vi "CODCr启动 (子VI).vi"(11 "元素":T1(ring)) -> (0 "error out":T2={"status"=FALSE, "代码"=4, "source"=""} caption="错误输出" {"代码" items=["执行成功"=1, "执行失败，但不知道原因"=2, "命令请求条件错误"=3, "通讯超时"=4, "系统繁忙不能执行"=5, "系统故障"=6, "没有数据"=100]})   [LabVIEW 2016]
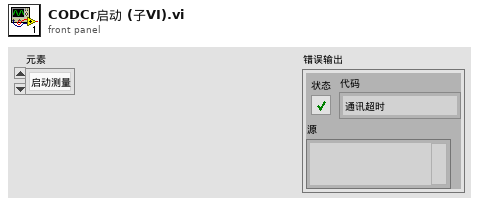
[diagram p1: front panel]
types:
  T1 = enum16{"启动测量", "标样核查", "零点核查", "跨度核查", "空白测试", "平行样测试", "加标回收", "空白校准", "标样校准", "初始化（清洗）", "停止测试", "仪器重启", "校时", "模式设置", "测量间隔设置"}
  T2 = cluster{"status":bool, "代码":u16, "source":string}
  T3 = cluster{"系统时间":timestamp, "工作状态":u16, "测量模式":u16, "告警代码":u16, "故障代码":u16, "日志代码":u16, "软件版本":u16, "F0":sgl, "F1":sgl, "F2":sgl, "F3":sgl, "T":sgl, "H":sgl, "id":u16, "flowid":u16, "量程":u16}
  T4 = cluster{"测量模式":enum16{"水样测量", "标样核查", "零点核查", "跨度核查", "空白测试", "加标回收", "平行样", "校零", "校标"}}
  T5 = enum16{"空闲", "水样测试", "标样核查", "零点核查", "跨度核查", "空白测试", "平行样测试", "加标回收", "空白校准", "标样校准", "初始化（清洗）"}
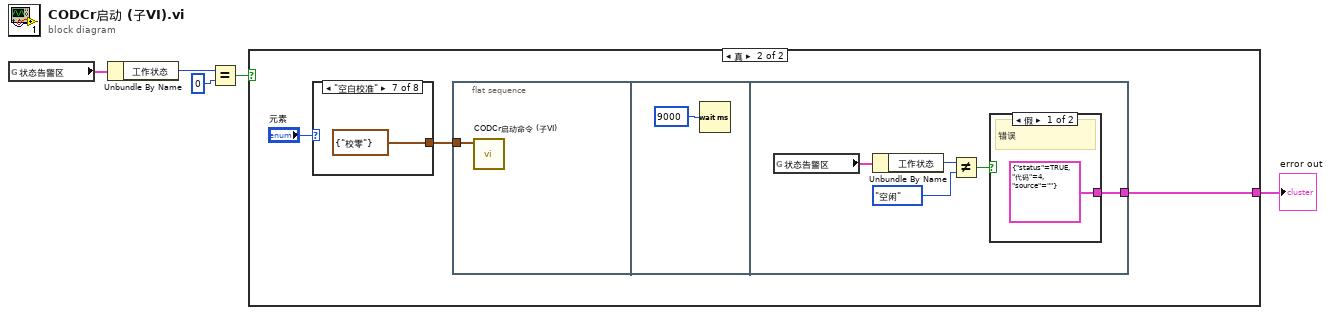
[diagram p0: block diagram]
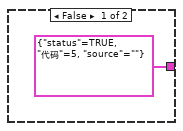
[diagram p2: hidden frame]
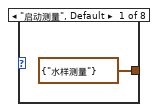
[diagram p3: hidden frame]
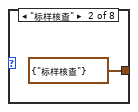
[diagram p4: hidden frame]
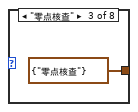
[diagram p5: hidden frame]
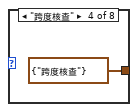
[diagram p6: hidden frame]
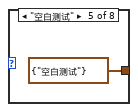
[diagram p7: hidden frame]
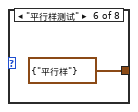
[diagram p8: hidden frame]
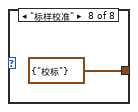
[diagram p9: hidden frame]
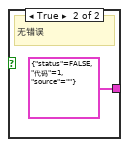
[diagram p10: hidden frame]
diagram:
  n1 = global read "CODcr全局变量.vi" "状态告警区"() -> (w1:T3)
  n2 = Unbundle By Name(w1) -> ("工作状态"=w5:u16)
  n3 = Equal?(x=w5, y=u16 0) -> (x = y?=w4:bool)
  n4 = case shown="真" w4 {
    tunnel: [T2 {"status"=TRUE, "代码"=5, "source"=""} ("error out") w9] -> w2
    frame False {
    }
    frame True {
      n5 = case shown="\"空白校准\"" "元素" {
        tunnel: [T4 {"测量模式"=enum."水样测量"} ("启动测量模式") T4 {"测量模式"=enum."标样核查"} ("启动测量模式") T4 {"测量模式"=enum."零点核查"} ("启动测量模式") T4 {"测量模式"=enum."跨度核查"} ("启动测量模式") T4 {"测量模式"=enum."空白测试"} ("启动测量模式") T4 {"测量模式"=enum."平行样"} ("启动测量模式") T4 {"测量模式"=enum."校零"} ("启动测量模式") T4 {"测量模式"=enum."校标"} ("启动测量模式")] -> w7
        frame "启动测量", Default {
        }
        frame "标样核查" {
        }
        frame "零点核查" {
        }
        frame "跨度核查" {
        }
        frame "空白测试" {
        }
        frame "平行样测试" {
        }
        frame "空白校准" {
        }
        frame "标样校准" {
        }
      }
      n6 = flat-sequence {
        tunnel: w7 -> [w18]
        tunnel: [w24] -> w9
        frame #0 {
          n7 = call "CODCr启动命令 (子VI).vi"("启动测量模式"=w18) -> ()  [unwired: 11 in]
        }
        frame #1 {
          n8 = Wait (ms)(milliseconds to wait=u32 9000 ("等待时间（毫秒）")) -> ()  [unwired: 1 out]
        }
        frame #2 {
          n9 = global read "CODcr全局变量.vi" "状态告警区"() -> (w20:T3)
          n10 = Unbundle By Name(w20) -> ("工作状态"=w22:u16)
          n11 = Not Equal?(x=w22, y=T5."空闲") -> (x != y?=w21:bool)
          n12 = case shown="假" w21 {
            tunnel: [T2 {"status"=TRUE, "代码"=4, "source"=""} ("error out") T2 {"status"=FALSE, "代码"=1, "source"=""} ("error out")] -> w24
            frame False {
              # "错误"
            }
            frame True {
              # "无错误"
            }
          }
        }
      }
    }
  }
  "error out" <- w2
